vi "CLSUIP_GetUnwiredTerminal.vi"(8 "error in (no error)":errorcluster, 11 "VI Refnum":refnum<vi>) -> (0 "error out":errorcluster, 1 "Multiframe Stuct out":refnum<vi>, 2 "Outer Terminal Ref":refnum<vi>, 3 "VI Refnum out":refnum<vi>)   [LabVIEW 2021, in "MemberVICreation.lvlib"]
uses:
  <resource>/Framework/Providers/LVClassLibrary/NewAccessors/MemberVICreation.lvlib
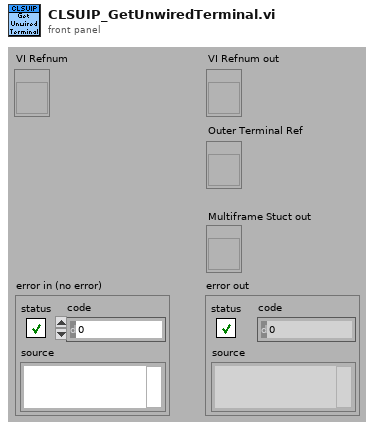
[diagram p1: front panel]
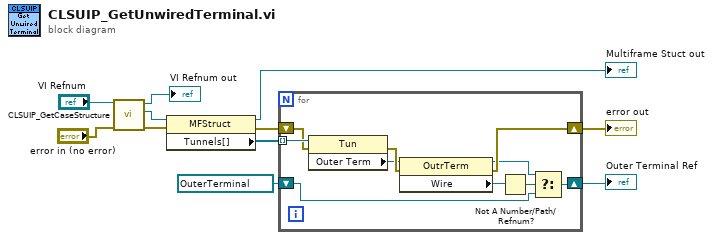
[diagram p0: block diagram]
diagram:
  n1 = call <resource>:"CLSUIP_GetCaseStructure.vi"("error in (no error)"="error in (no error)", "VI Refnum"="VI Refnum") -> ("error out"=w8:errorcluster, "CaseStructure Ref"=w7:refnum<vi>, "VI Refnum out"=→"VI Refnum out":refnum<vi>)  [unwired: 7 out]
  n2 = property class="MFStruct"(reference=w7, error in=w8) -> (reference out=→"Multiframe Stuct out":refnum<vi>, error out=w5:errorcluster, "Tunnels[]"=w6:refnum<vi>[])
  n3 = for {
    tunnel: w6 -> [w21] mode=indexing
    shift-right: [w15] -> w2
    shift-left: w5 -> [w20]
    shift-right: [w13] -> w3
    shift-left: refnum<vi> refnum ("Outer Term") -> [w12]
    n4 = property class="Tun"(reference=w21, error in=w20) -> (error out=w19:errorcluster, "Outer Term"=w18:refnum<vi>)  [unwired: 1 out]
    n5 = property class="OutrTerm"(reference=w18, error in=w19) -> (reference out=w14:refnum<vi>, error out=w15:errorcluster, "Wire"=w17:refnum<vi>)
    n6 = Not A Number/Path/Refnum?(number/path/refnum=w17) -> (NaN/Path/Refnum?=w16:bool)
    n7 = Select(t=w14, s=w16, f=w12) -> (s? t:f=w13:refnum<vi>)
  }
  "error out" <- w2
  "Outer Terminal Ref" <- w3
